vi "ASSIGN_opc.vi"() -> ()   [LabVIEW 2020]
panel:
  out "[COMP_PRESENT_STATUS]":i32
  out "[PRE_PRESSURE_STATUS]":i32
  out "[INBOARD_LOAD_MIN]":dbl
  out "[INBOARD_LOAD]":dbl
  out "[INBOARD_LOAD_MAX]":dbl
  out "[OUTBOARD_LOAD_MIN]":dbl
  out "[OUTBOARD_LOAD]":dbl
  out "[OUTBOARD_LOAD_MAX]":dbl
  out "[LOAD_CHK_STATUS]":i32
  out "[PROFILE_CHK_STATUS]":i32
  out "[VISION_CHK_STATUS]":i32
  out "[MARKING_TEXT]":string
  out "[MARKING_STATUS]":i32
  out "[CT]":dbl
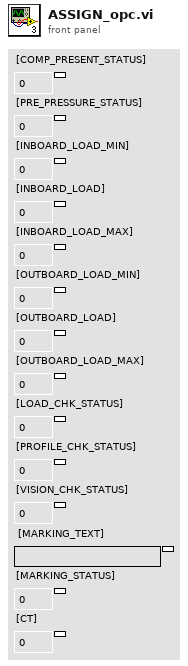
[diagram p1: front panel]
types:
  T1 = enum32{"No DataSocket", "Publish", "Subscribe", "Publish & Subscribe"}
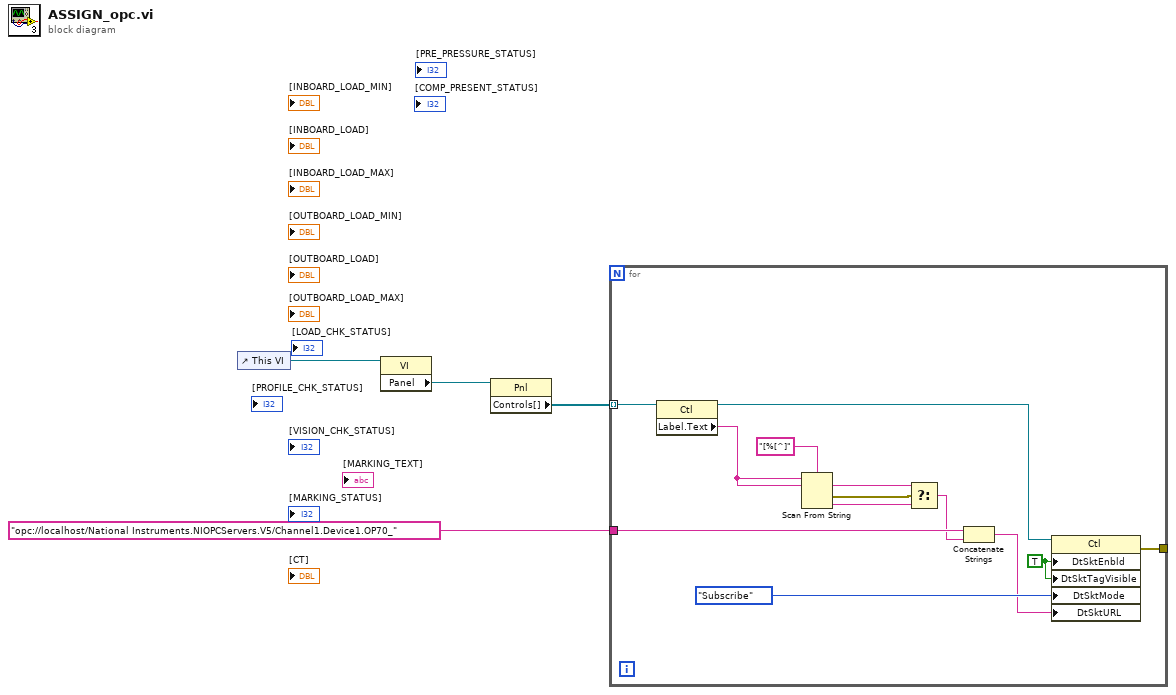
[diagram p0: block diagram]
diagram:
  n1 = control-ref of="This VI"() -> (w4:refnum<vi>)
  n2 = property class="VI"(reference=w4) -> ("Panel"=w3:refnum<vi>)  [unwired: 1 in, 2 out]
  n3 = property class="Pnl"(reference=w3) -> ("Controls[]"=w2:refnum<vi>[])  [unwired: 1 in, 2 out]
  n4 = for {
    tunnel: w2 -> [w16] mode=indexing
    tunnel: "opc://localhost/National Instruments.NIOPCServers.V5/Channel1.Device1.OP70_" ("DataSocket:URL") -> [w9]
    tunnel: [w5] -> _
    w11 = TRUE ("DataSocket:Enabled")
    n5 = property class="Ctl"(reference=w16) -> (reference out=w6:refnum<vi>, "Label.Text"=w13:string)  [unwired: 1 in, 1 out]
    n6 = Scan From String(format string="[%[^]", input string=w13) -> (error out=w14:errorcluster, output 1=w12:string)  [unwired: 3 in, 2 out]
    n7 = Select(t=w13, s=w14, f=w12) -> (s? t:f=w8:string)
    n8 = Concatenate Strings(w9, w8) -> (w7:string)
    n9 = property on="Property Node" class="Ctl"(reference=w6, "DtSktEnbld"=w11, "DtSktTagVisible"=w11, "DtSktMode"=T1."Subscribe" ("DataSocket:Mode"), "DtSktURL"=w7) -> (error out=w5:errorcluster)  [unwired: 1 in, 1 out]
  }
